vi "GPIO Pins to String.vi"(10 "Result Pins":i32[](array[ring]) items=["EXT1"=1, "EXT2"=2, "EXT3"=3, "EXT4"=4, "EXT5"=5, "EXT6"=6, "EXT7"=7]) -> (2 "Result String":string)   [LabVIEW 2012, in "Keysight B2980 Series.lvlib"]
doc: "Parse GPIO Pins array into a comma separated string which can be recognized by SCPI commads."
uses:
  Keysight B2980 Series.lvlib
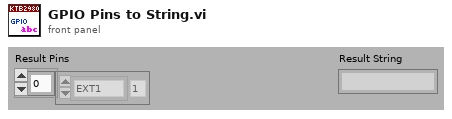
[diagram p1: front panel]
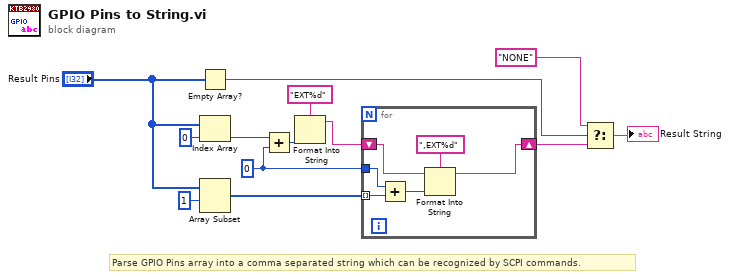
[diagram p0: block diagram]
diagram:
  w4 = 0 ("y")
  # "Parse GPIO Pins array into a comma separated string which can be recognized by SCPI commands."
  n1 = Empty Array?(array="Result Pins") -> (empty?=w13:bool)
  n2 = Index Array(array="Result Pins", index=0) -> (element=w5:i32)
  n3 = Array Subset(array="Result Pins", index=1) -> (w11:i32[])  [unwired: 1 in]
  n4 = Add(x=w5, y=w4) -> (x+y=w6:i32)
  n5 = Format Into String(format string="EXT%d", w6) -> (resulting string=w7:string)  [unwired: 2 in, 1 out]
  n6 = for {
    tunnel: w11 -> [w17] mode=indexing
    shift-right: [w14] -> w3
    shift-left: w7 -> [w15]
    tunnel: w4 -> [w16]
    n7 = Add(x=w16, y=w17) -> (x+y=w18:i32)
    n8 = Format Into String(format string=",EXT%d", initial string=w15, w18) -> (resulting string=w14:string)  [unwired: 1 in, 1 out]
  }
  n9 = Select(t="NONE", s=w13, f=w3) -> (s? t:f=→"Result String":string)
